vi "输出文本.vi"(10 "当前档位":string, 11 "字符串":string) -> (3 "输出文本":string)   [LabVIEW 2016]
panel:
  out "子字符串;substring 2":string
  out "子字符串;substring":string
  out "Elapsed Time Text":string caption="已用时间文本"
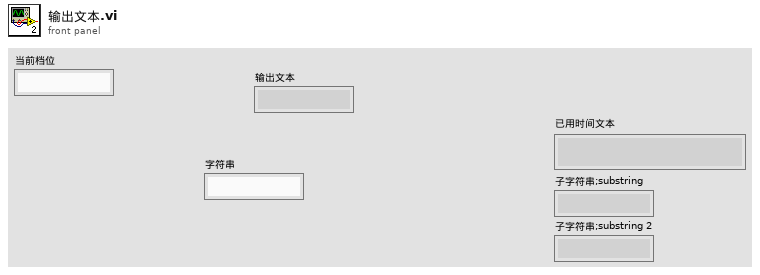
[diagram p1: front panel]
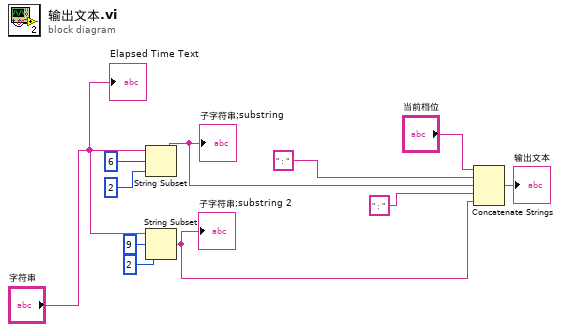
[diagram p0: block diagram]
diagram:
  n1 = String Subset(string="字符串", offset (0)=6 ("偏移量(0)"), length (rest)=2 ("长度（剩余）")) -> (substring=w5:string)
  "子字符串;substring" <- w5
  n2 = String Subset(string="字符串", offset (0)=9 ("偏移量(0)"), length (rest)=2 ("长度（剩余）")) -> (substring=w6:string)
  "子字符串;substring 2" <- w6
  n3 = Concatenate Strings("当前档位", "：", w5, "：" ("字符串"), w6) -> (→"输出文本":string)
  "Elapsed Time Text" <- "字符串"
